vi "HardwareConfiguration.vi"() -> (3 "configured?":bool)   [LabVIEW 2013]
uses:
  InstrControl/InstrumentSetup.vi
  globals/QC_RunInformation.vi
  InstrControl/InstrControl.lvclass
panel:
  in  "Matrix Configurations":bool
  in  "Defaults Multimeter":bool
  in  "Multimeter":enum32{"Keithley 2000"}(tab)
  in  "Range Value\n(0.1 - 100)":dbl=100.0 format="%#.2g"
  in  "Range":u16(ring) items=["Auto", "Manual"]
  in  "Function":u16(ring)=3 items=["AC Current", "DC Current", "AC Voltage", "DC Voltage", "2W-Resistance", "4W-Resistance", "Period", "Frequency", "Temperature", "Diode", "Continuity"]
  in  "Address KE2000":refnum<visa-resource-name>
  in  "Defaults LCR":bool
  in  "LCRs":enum32{"WayneKerr 6440B", "WayneKerr 6425"}(tab)
  in  "AC frequency [Hz]":i32=1000 format="%#.3p"
  in  "RC Configuration":u16(ring) items=["serial", "parallel"]
  in  "AC amplitude [V]":sgl=0.1
  in  "Address WK6440B":refnum<visa-resource-name>
  in  "Address WK6425":refnum<visa-resource-name>
  in  "AC amplitude [V] WK6425":sgl=0.1 caption="AC amplitude [V]"
  in  "RC Configuration WK6425":u16(ring) caption="RC Configuration" items=["serial", "parallel"]
  in  "AC frequency [Hz] WK6425":i32=1000 caption="AC frequency [Hz]" format="%#.3p"
  in  "VISA address":refnum<visa-resource-name>="COM24" caption="Arduino address"
  out "Programm uploaded?":string="Make sure programme is uploaded to Arduino Uno ->"
  in  "Blank Button":bool
  in  "Supplies":T1(tab)
  in  "Current Limit [µA]":sgl=100.0
  in  "Address KE2410":refnum<visa-resource-name>
  in  "Address KE487":refnum<visa-resource-name>
  in  "Compliance":u16(ring) items=["20µA", "2mA"]
  in  "Range:":u16(ring) items=["Autorange", "2nA", "20nA", "200nA", "2 microAmp", "20 microAmp", "200 microAmp", "2 milliAmp"]
  in  "Current Limit":u16(ring)=1 items=["OFF", "ON"]
  in  "Address KE6517":refnum<visa-resource-name>
  in  "current compliance \nlevel [mA]":dbl=0.0001 format="%.4f"
  in  "compliance/measurement\nrange (auto:0)":u16(ring)=6 items=["auto / auto", "1 nA / 1.1 V", "10 nA / 11 V", "100 nA / 110 V", "0.001 mA / 110 V", "0.01 mA / 110 V", "0.1 mA / 110 V", "1 mA / 110 V", "10 mA / 110 V", "100 mA / 110 V"]
  in  "Address KE236":refnum<visa-resource-name>
  in  "Defaults Supply":bool
  in  "OK Button":bool
  # "Hardware Configuration"
  # "Multimeter Configuration"
  # "Supply Configuration"
  # "Arduino Configuration"
  # "LCR Configuration"
  # "(Only for initialisation)"
  # "(Only for initialisation)"
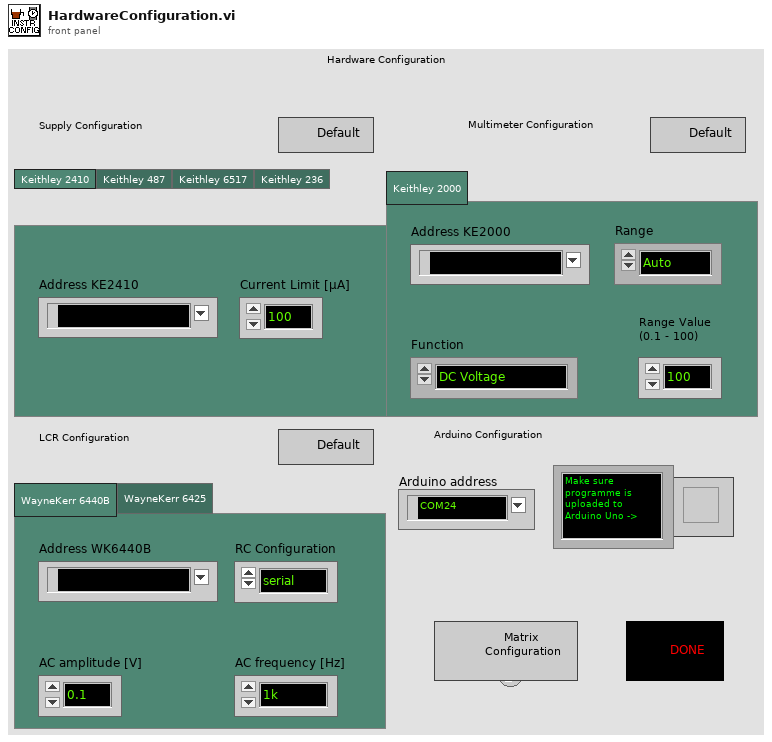
[diagram p1: front panel]
types:
  T1 = enum32{"Keithley 2410", "Keithley 487", "Keithley 6517", "Keithley 236"}
  T2 = cluster{"KE 2410":cluster{"Instrument name":string, "address":refnum<visa-resource-name>, "Instrument type":u16}, "KE 6517":cluster{"Instrument name":string, "address":refnum<visa-resource-name>, "Instrument type":u16}, "KE 487":cluster{"Instrument name":string, "address":refnum<visa-resource-name>, "Instrument type":u16}, "KE 236":cluster{"Instrument name":string, "address":refnum<visa-resource-name>, "Instrument type":u16}, "WK 6440B":cluster{"Instrument name":string, "address":refnum<visa-resource-name>, "Instrument type":u16}, "WK 6425":cluster{"Instrument name":string, "address":refnum<visa-resource-name>, "Instrument type":u16}, "Pickering Matrix":cluster{"Instrument name":string, "address":refnum<visa-resource-name>, "Instrument type":u16}, "KE 2000":cluster{"Instrument name":string, "address":refnum<visa-resource-name>, "Instrument type":u16}, "KE3706A Switching":cluster{"Instrument name":string, "address":refnum<visa-resource-name>, "Instrument type":u16}}
  T3 = cluster{"VISA address":refnum<visa-resource-name>, "T sensor":enum16{"SHT", "DS"}, "Arduino":refnum<class "ArduinoControl.lvclass">}
  T4 = cluster{"Range":u16, "Range Value":dbl, "Function":u16, "KE2000":refnum<class "KE2000.lvclass">}
  T5 = cluster{"Current Limit":sgl, "KE2410":refnum<class "KE2410.lvclass">}
  T6 = cluster{"Compliance":u16, "Range:":u16, "KE487":refnum<class "KE487.lvclass">}
  T7 = cluster{"Current Limit":u16, "KE6517":refnum<class "KE6517.lvclass">}
  T8 = cluster{"current \ncompliance level":dbl, "compliance/\nmeasurement range (auto:0)":u16, "KE236":refnum<class "KE236.lvclass">}
  T9 = cluster{"Sensor Serial No.:":string, "Wafer Serial No.:":string, "Batch:":string, "Manufacturer:":string, "Device Category:":string, "Database Serial No.:":string, "Date Initiated:":string, "Time Initiated:":string, "Test":string, "Instruments used:":string, "Probeplan used:":string, "End of Run comment:":string, "User:":string}
  T10 = cluster{"RC Configuration":u16, "AC amplitude [V]":dbl, "AC frequency [Hz]":i32, "WK6440B":refnum<class "WK6440B.lvclass">}
  T11 = cluster{"RC Configuration":u16, "AC amplitude [V]":dbl, "AC frequency [Hz]":i32, "WK6425":refnum<class "WK6425.lvclass">}
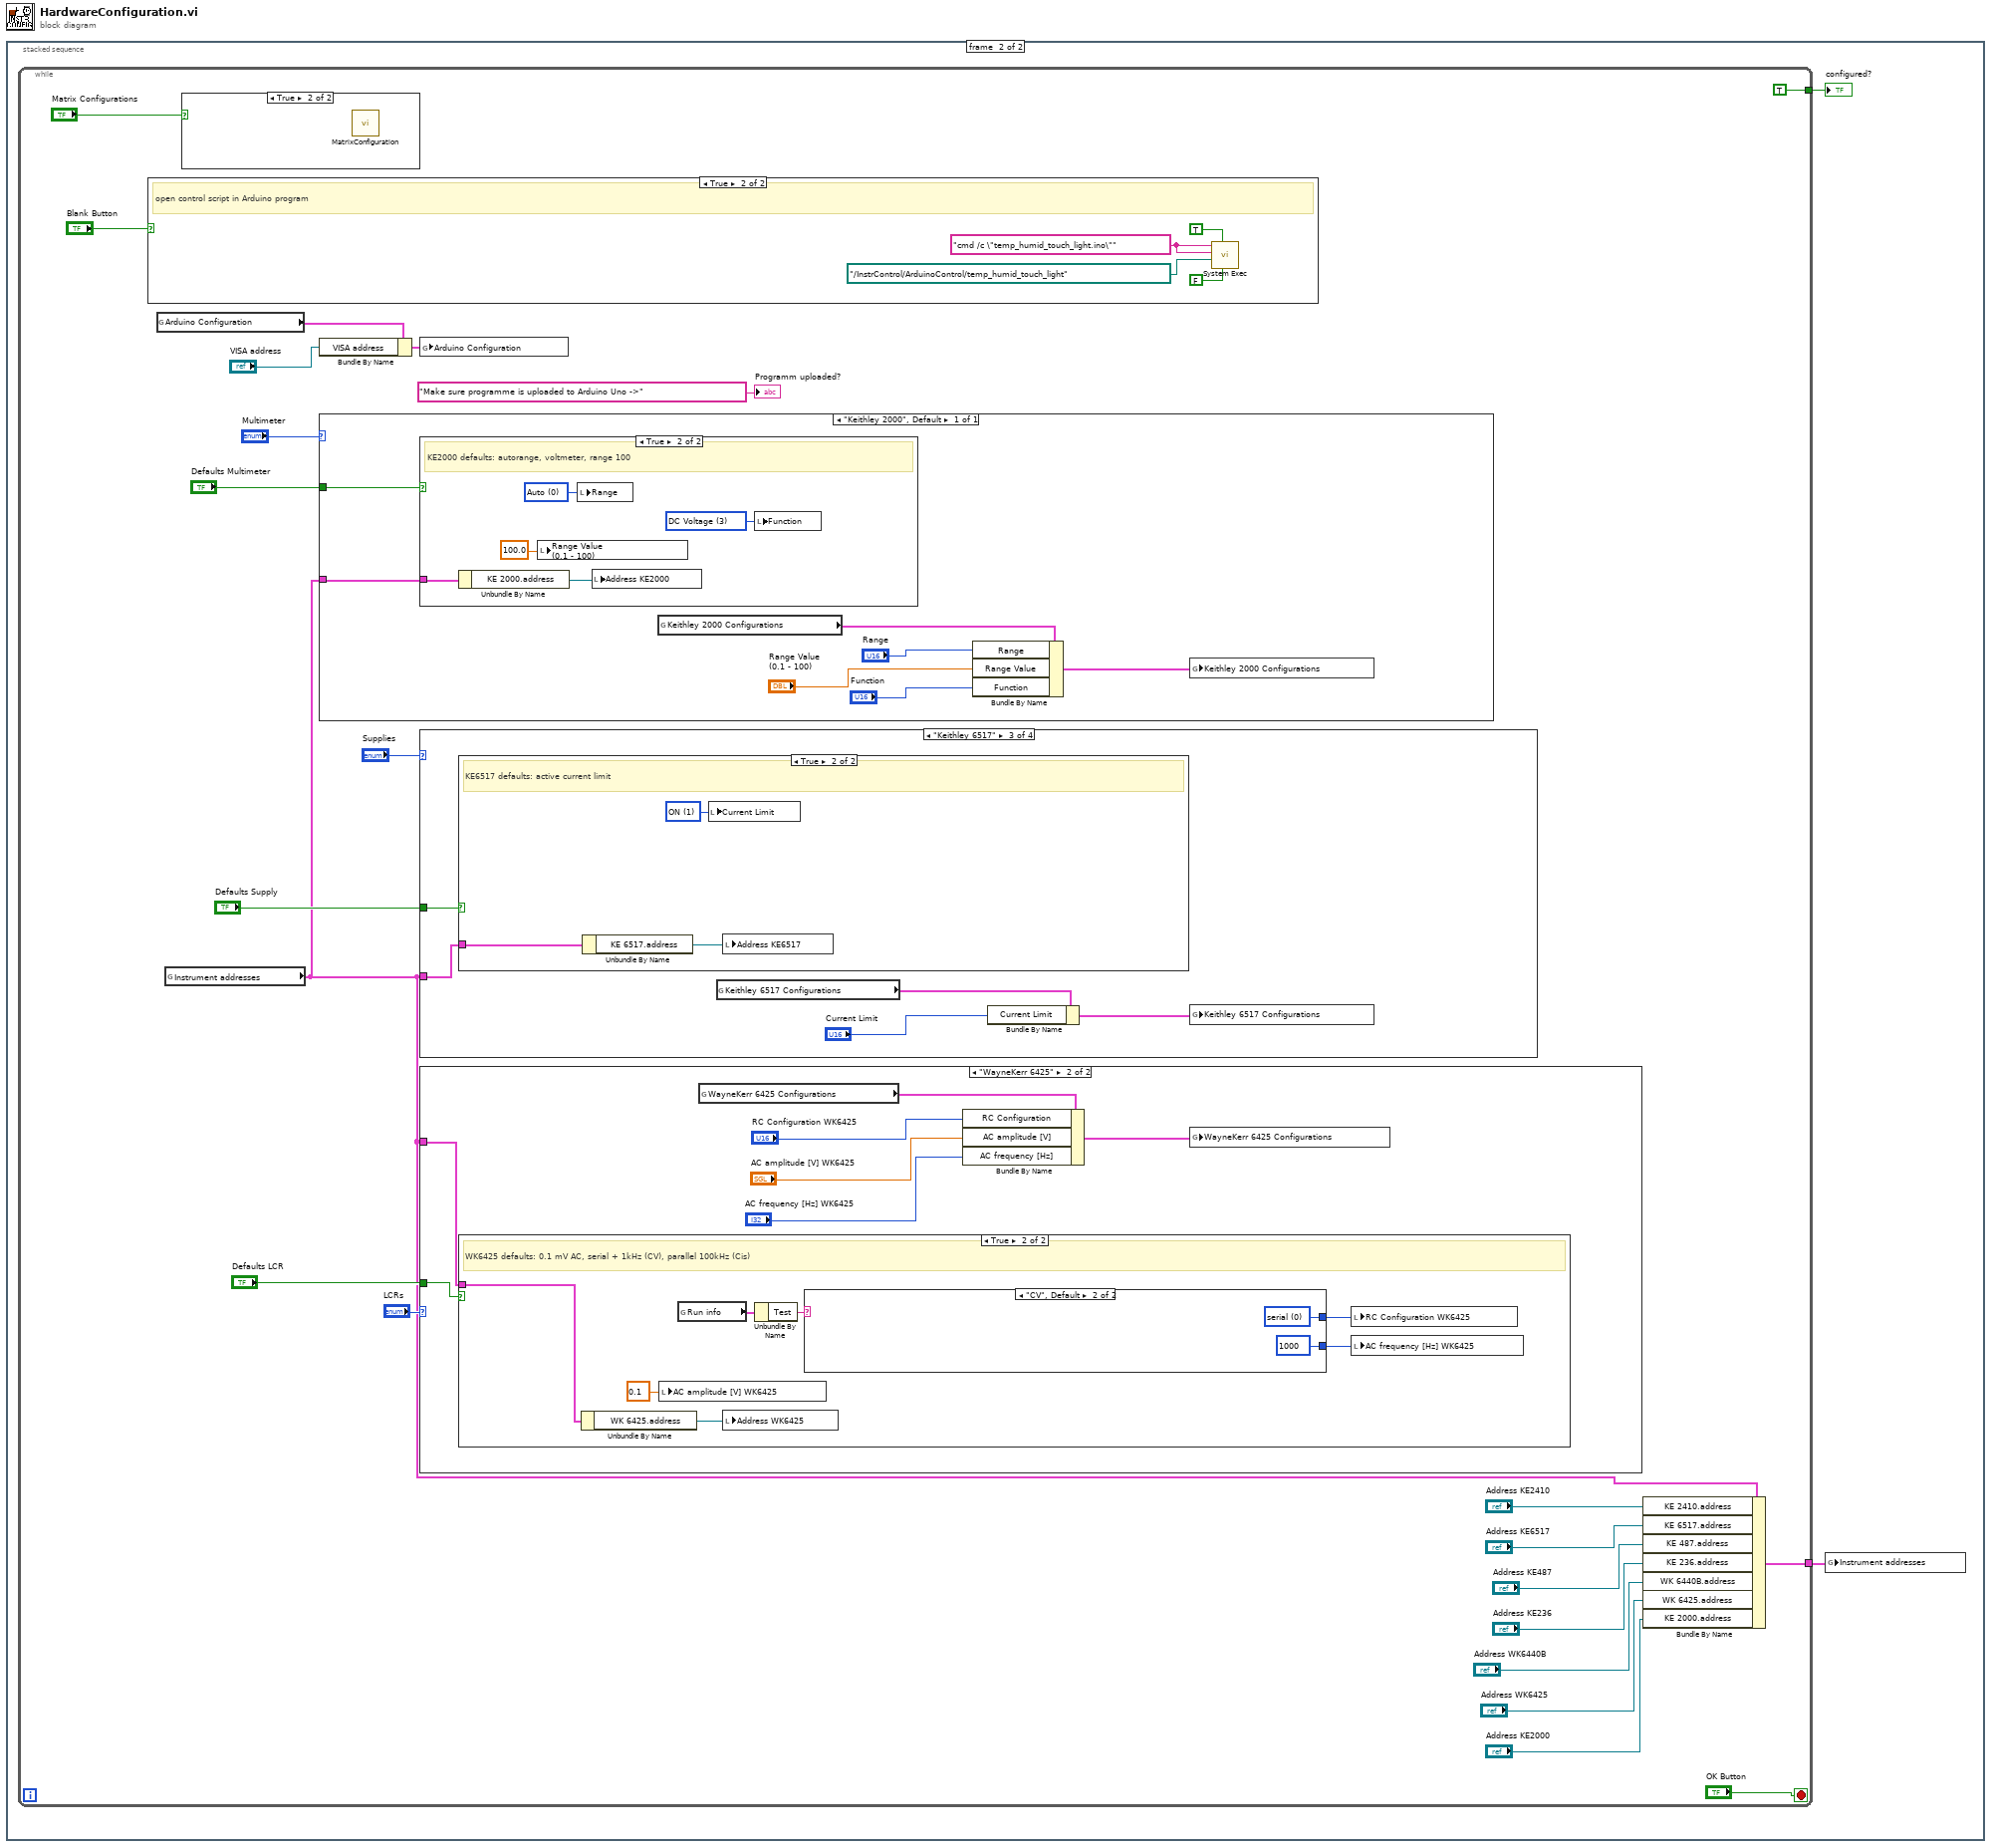
[diagram p0: block diagram]
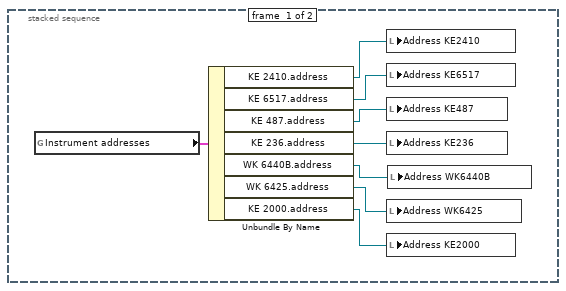
[diagram p2: hidden frame]
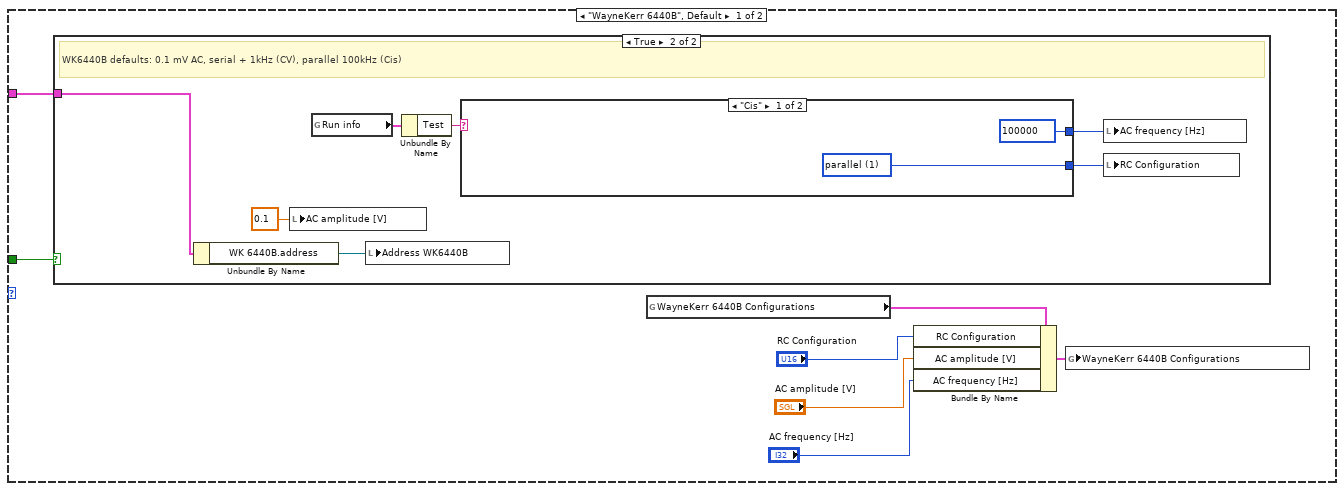
[diagram p6: hidden frame]
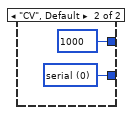
[diagram p8: hidden frame]
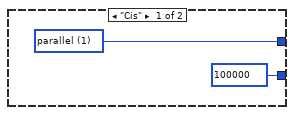
[diagram p10: hidden frame]
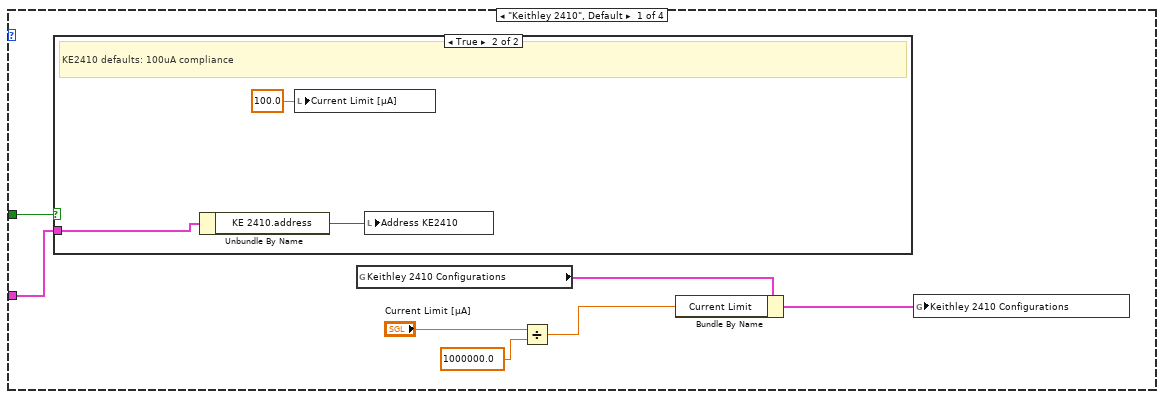
[diagram p11: hidden frame]
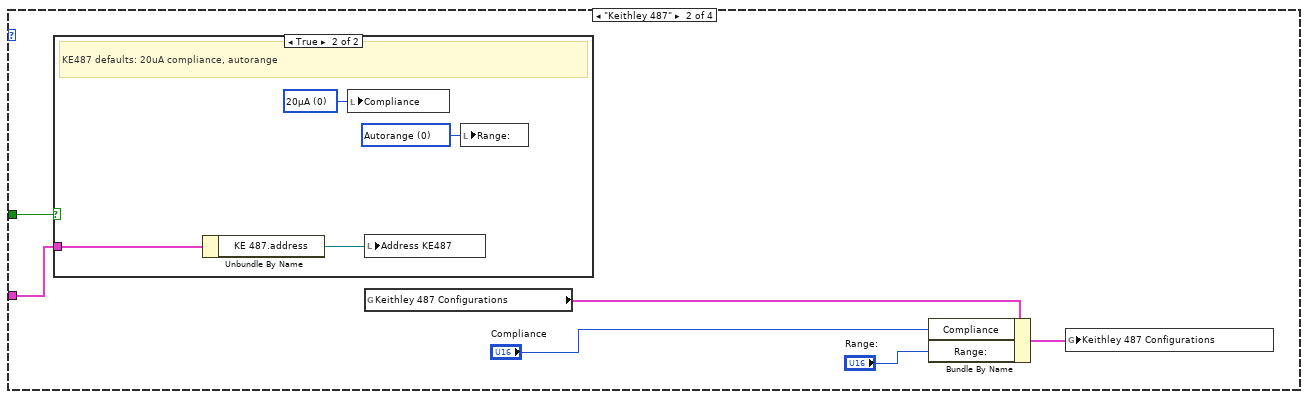
[diagram p13: hidden frame]
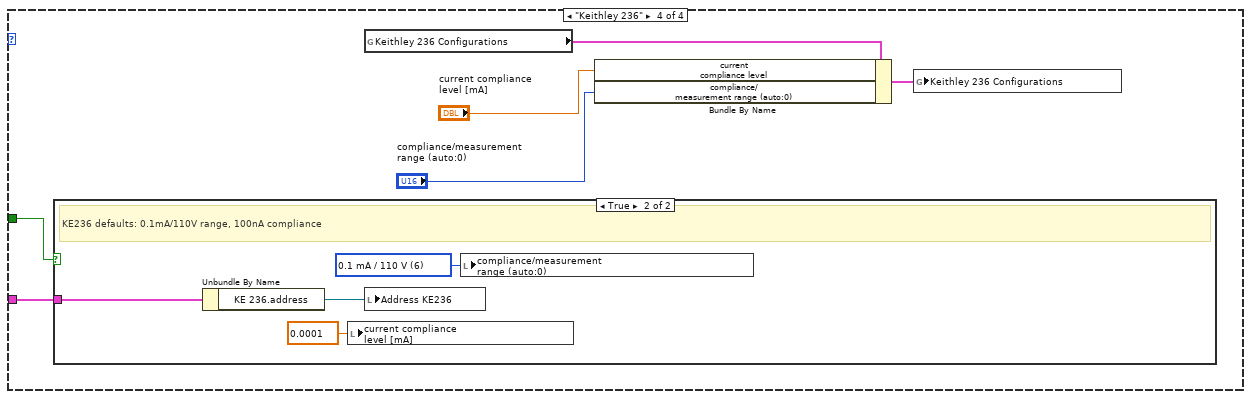
[diagram p16: hidden frame]
diagram:
  n1 = stacked-sequence {
    frame #0 {
      n2 = global read "InstrumentSetup.vi" "Instrument addresses"() -> (w8:T2)
      n3 = Unbundle By Name(w8) -> ("KE 2410.address"=w7:refnum<visa-resource-name>, "KE 6517.address"=w6:refnum<visa-resource-name>, "KE 487.address"=w5:refnum<visa-resource-name>, "KE 236.address"=w4:refnum<visa-resource-name>, "WK 6440B.address"=w3:refnum<visa-resource-name>, "WK 6425.address"=w2:refnum<visa-resource-name>, "KE 2000.address"=w1:refnum<visa-resource-name>)
      n4 = local write "Address KE2410"(w7) -> ()
      n5 = local write "Address KE6517"(w6) -> ()
      n6 = local write "Address KE487"(w5) -> ()
      n7 = local write "Address KE236"(w4) -> ()
      n8 = local write "Address WK6425"(w2) -> ()
      n9 = local write "Address KE2000"(w1) -> ()
      n10 = local write "Address WK6440B"(w3) -> ()
    }
    frame #1 {
      n11 = while {
        tunnel: [TRUE] -> w10
        tunnel: [w17] -> w9
        stop <- "OK Button" stop-if-true
        n12 = case shown="True" "Blank Button" {
          frame False {
          }
          frame True {
            w35 = "cmd /c \"temp_humid_touch_light.ino\""
            # "open control script in Arduino program"
            n13 = call <vilib>:"System Exec.vi"("run minimized? (F)"=FALSE, "wait until completion? (T)"=TRUE, "working directory"=path "../InstrControl/ArduinoControl/temp_humid_touch_light", "standard input"=w35, "command line"=w35) -> ()  [unwired: 3 in, 4 out]
          }
        }
        n14 = global read "InstrumentSetup.vi" "Arduino Configuration"() -> (w24:T3)
        n15 = global read "InstrumentSetup.vi" "Instrument addresses"() -> (w19:T2)
        n16 = case shown="True" "Matrix Configurations" {
          frame False {
          }
          frame True {
            n17 = call "MatrixConfiguration.vi"() -> ()  [unwired: 12 in]
          }
        }
        n18 = Bundle By Name(cluster=w24, "VISA address"="VISA address") -> (w23:T3)
        n19 = case shown="\"Keithley 2000\", Default" "Multimeter" {
          tunnel: "Defaults Multimeter" -> [w44]
          tunnel: w19 -> [w41]
          frame "Keithley 2000", Default {
            n20 = case shown="True" w44 {
              tunnel: w41 -> [_ w49]
              frame False {
              }
              frame True {
                w47 = u16 0 items=["Auto", "Manual"] ("Range")
                w48 = u16 3 items=["AC Current", "DC Current", "AC Voltage", "DC Voltage", "2W-Resistance", "4W-Resistance", "Period", "Frequency", "Temperature", "Diode", "Continuity"] ("Function")
                # "KE2000 defaults: autorange, voltmeter, range 100"
                n21 = Unbundle By Name(w49) -> ("KE 2000.address"=w45:refnum<visa-resource-name>)
                n22 = local write "Range Value\n(0.1 - 100)"(100.0 ("Range Value\n(0.1 - 100)")) -> ()
                n23 = local write "Range"(w47) -> ()
                n24 = local write "Address KE2000"(w45) -> ()
                n25 = local write "Function"(w48) -> ()
              }
            }
            n26 = global read "InstrumentSetup.vi" "Keithley 2000 Configurations"() -> (w43:T4)
            n27 = Bundle By Name(cluster=w43, "Range"="Range", "Range Value"="Range Value\n(0.1 - 100)", "Function"="Function") -> (w42:T4)
            n28 = global write "InstrumentSetup.vi" "Keithley 2000 Configurations"(w42) -> ()
          }
        }
        n29 = global write "InstrumentSetup.vi" "Arduino Configuration"(w23) -> ()
        n30 = case shown="\"Keithley 6517\"" "Supplies" {
          tunnel: "Defaults Supply" -> [w92 w101 w110 w119]
          tunnel: w19 -> [w87 w98 w107 w116]
          frame "Keithley 2410", Default {
            n31 = case shown="True" w92 {
              tunnel: w87 -> [_ w95]
              frame False {
              }
              frame True {
                # "KE2410 defaults: 100uA compliance"
                n32 = Unbundle By Name(w95) -> ("KE 2410.address"=w93:refnum<visa-resource-name>)
                n33 = local write "Current Limit [µA]"(100.0) -> ()
                n34 = local write "Address KE2410"(w93) -> ()
              }
            }
            n35 = global read "InstrumentSetup.vi" "Keithley 2410 Configurations"() -> (w91:T5)
            n36 = Divide(x="Current Limit [µA]", y=1000000.0) -> (x/y=w88:dbl)
            n37 = Bundle By Name(cluster=w91, "Current Limit"=w88) -> (w90:T5)
            n38 = global write "InstrumentSetup.vi" "Keithley 2410 Configurations"(w90) -> ()
          }
          frame "Keithley 487" {
            n39 = case shown="True" w101 {
              tunnel: w98 -> [_ w105]
              frame False {
              }
              frame True {
                w103 = u16 0 items=["Autorange", "2nA", "20nA", "200nA", "2 microAmp", "20 microAmp", "200 microAmp", "2 milliAmp"] ("Range:")
                w104 = u16 0 items=["20µA", "2mA"] ("Compliance")
                # "KE487 defaults: 20uA compliance, autorange"
                n40 = Unbundle By Name(w105) -> ("KE 487.address"=w102:refnum<visa-resource-name>)
                n41 = local write "Compliance"(w104) -> ()
                n42 = local write "Address KE487"(w102) -> ()
                n43 = local write "Range:"(w103) -> ()
              }
            }
            n44 = global read "InstrumentSetup.vi" "Keithley 487 Configurations"() -> (w100:T6)
            n45 = Bundle By Name(cluster=w100, "Compliance"="Compliance", "Range:"="Range:") -> (w99:T6)
            n46 = global write "InstrumentSetup.vi" "Keithley 487 Configurations"(w99) -> ()
          }
          frame "Keithley 6517" {
            n47 = case shown="True" w110 {
              tunnel: w107 -> [_ w113]
              frame False {
              }
              frame True {
                w112 = u16 1 items=["OFF", "ON"] ("Current Limit")
                # "KE6517 defaults: active current limit"
                n48 = Unbundle By Name(w113) -> ("KE 6517.address"=w111:refnum<visa-resource-name>)
                n49 = local write "Current Limit"(w112) -> ()
                n50 = local write "Address KE6517"(w111) -> ()
              }
            }
            n51 = global read "InstrumentSetup.vi" "Keithley 6517 Configurations"() -> (w109:T7)
            n52 = Bundle By Name(cluster=w109, "Current Limit"="Current Limit") -> (w108:T7)
            n53 = global write "InstrumentSetup.vi" "Keithley 6517 Configurations"(w108) -> ()
          }
          frame "Keithley 236" {
            n54 = case shown="True" w119 {
              tunnel: w116 -> [_ w123]
              frame False {
              }
              frame True {
                w121 = u16 6 items=["auto / auto", "1 nA / 1.1 V", "10 nA / 11 V", "100 nA / 110 V", "0.001 mA / 110 V", "0.01 mA / 110 V", "0.1 mA / 110 V", "1 mA / 110 V", "10 mA / 110 V", "100 mA / 110 V"] ("compliance/\nmeasurement range (auto:0)")
                # "KE236 defaults: 0.1mA/110V range, 100nA compliance"
                n55 = Unbundle By Name(w123) -> ("KE 236.address"=w120:refnum<visa-resource-name>)
                n56 = local write "current compliance \nlevel [mA]"(0.0001 ("current \ncompliance level")) -> ()
                n57 = local write "Address KE236"(w120) -> ()
                n58 = local write "compliance/measurement\nrange (auto:0)"(w121) -> ()
              }
            }
            n59 = global read "InstrumentSetup.vi" "Keithley 236 Configurations"() -> (w117:T8)
            n60 = Bundle By Name(cluster=w117, "current \ncompliance level"="current compliance \nlevel [mA]", "compliance/\nmeasurement range (auto:0)"="compliance/measurement\nrange (auto:0)") -> (w118:T8)
            n61 = global write "InstrumentSetup.vi" "Keithley 236 Configurations"(w118) -> ()
          }
        }
        n62 = case shown="\"WayneKerr 6425\"" "LCRs" {
          tunnel: "Defaults LCR" -> [w54 w72]
          tunnel: w19 -> [w53 w71]
          frame "WayneKerr 6440B", Default {
            n63 = case shown="True" w54 {
              tunnel: w53 -> [_ w63]
              frame False {
              }
              frame True {
                # "WK6440B defaults: 0.1 mV AC, serial + 1kHz (CV), parallel 100kHz (Cis)"
                n64 = Unbundle By Name(w63) -> ("WK 6440B.address"=w57:refnum<visa-resource-name>)
                n65 = local write "AC amplitude [V]"(0.1) -> ()
                n66 = global read "QC_RunInformation.vi" "Run info"() -> (w59:T9)
                n67 = local write "Address WK6440B"(w57) -> ()
                n68 = Unbundle By Name(w59) -> ("Test"=w58:string)
                n69 = case shown="\"Cis\"" w58 {
                  tunnel: [w65 w67] -> w61
                  tunnel: [100000 1000] -> w60
                  frame "Cis" {
                    w65 = u16 1 items=["serial", "parallel"] ("RC Configuration")
                  }
                  frame "CV", Default {
                    w67 = u16 0 items=["serial", "parallel"] ("RC Configuration")
                  }
                }
                n70 = local write "AC frequency [Hz]"(w60) -> ()
                n71 = local write "RC Configuration"(w61) -> ()
              }
            }
            n72 = global read "InstrumentSetup.vi" "WayneKerr 6440B Configurations"() -> (w56:T10)
            n73 = Bundle By Name(cluster=w56, "RC Configuration"="RC Configuration", "AC amplitude [V]"="AC amplitude [V]", "AC frequency [Hz]"="AC frequency [Hz]") -> (w55:T10)
            n74 = global write "InstrumentSetup.vi" "WayneKerr 6440B Configurations"(w55) -> ()
          }
          frame "WayneKerr 6425" {
            n75 = case shown="True" w72 {
              tunnel: w71 -> [_ w81]
              frame False {
              }
              frame True {
                # "WK6425 defaults: 0.1 mV AC, serial + 1kHz (CV), parallel 100kHz (Cis)"
                n76 = Unbundle By Name(w81) -> ("WK 6425.address"=w75:refnum<visa-resource-name>)
                n77 = local write "AC amplitude [V] WK6425"(0.1) -> ()
                n78 = global read "QC_RunInformation.vi" "Run info"() -> (w77:T9)
                n79 = local write "Address WK6425"(w75) -> ()
                n80 = Unbundle By Name(w77) -> ("Test"=w76:string)
                n81 = case shown="\"CV\", Default" w76 {
                  tunnel: [w83 w85] -> w79
                  tunnel: [100000 1000] -> w78
                  frame "Cis" {
                    w83 = u16 1 items=["serial", "parallel"] ("RC Configuration")
                  }
                  frame "CV", Default {
                    w85 = u16 0 items=["serial", "parallel"] ("RC Configuration")
                  }
                }
                n82 = local write "RC Configuration WK6425"(w79) -> ()
                n83 = local write "AC frequency [Hz] WK6425"(w78) -> ()
              }
            }
            n84 = global read "InstrumentSetup.vi" "WayneKerr 6425 Configurations"() -> (w74:T11)
            n85 = Bundle By Name(cluster=w74, "RC Configuration"="RC Configuration WK6425", "AC amplitude [V]"="AC amplitude [V] WK6425", "AC frequency [Hz]"="AC frequency [Hz] WK6425") -> (w73:T11)
            n86 = global write "InstrumentSetup.vi" "WayneKerr 6425 Configurations"(w73) -> ()
          }
        }
        n87 = Bundle By Name(cluster=w19, "KE 2410.address"="Address KE2410", "KE 6517.address"="Address KE6517", "KE 487.address"="Address KE487", "KE 236.address"="Address KE236", "WK 6440B.address"="Address WK6440B", "WK 6425.address"="Address WK6425", "KE 2000.address"="Address KE2000") -> (w17:T2)
        "Programm uploaded?" <- "Make sure programme is uploaded to Arduino Uno ->"
      }
      "configured?" <- w10
      n88 = global write "InstrumentSetup.vi" "Instrument addresses"(w9) -> ()
    }
  }
